vi "Begin.vi"(8 "error in":errorcluster) -> (0 "error out":errorcluster)   [LabVIEW 2019]
doc: "Called before other user functions, this VI is expected to open initial I/O refnums, load in file data, and do all program initialization. Notice that the <B>error out</B> terminal is simply used for data flow. Wiring it to other structures or subVIs ensures that this VI runs first."
uses:
  <vilib>/Rock Robotics/WPI/DriverStation/WPI_DriverStationRobotMode2.ctl
  <vilib>/Rock Robotics/WPI/Joystick/WPI_JoystickDeviceEnum.ctl
  <vilib>/Rock Robotics/WPI/Solenoid/WPI_SolenoidChannel.ctl
  <vilib>/Rock Robotics/SystemInterfaces/spilib/spi_bus.ctl
  <vilib>/Rock Robotics/WPI/ThirdParty/Phoenix-LabVIEW/Motor Controller/Controls/CTRE_Phoenix_MotorControl_NeutralMode.ctl
  <vilib>/Playing With Fusion Inc/Playing With Fusion Lib for FRC/PWF_ToF_LabVIEW/Public/TypeDefs/PwF_ToF_RangingMode.ctl
  <vilib>/Rock Robotics/WPI/ThirdParty/Phoenix-LabVIEW/Motor Controller/Controls/CTRE_Phoenix_MotorControl_ControlMode.ctl
  <vilib>/Rock Robotics/SystemInterfaces/i2clib/i2c_bus.ctl
  Robot Global Data.vi
  <vilib>/Rock Robotics/Network Tables/NT Write String Array.vi
  <vilib>/Rock Robotics/Network Tables/NT Read Number.vi
  <vilib>/Rock Robotics/WPI/Solenoid/WPI_SolenoidOpenSingle.vi
  <vilib>/Rock Robotics/WPI/Gyro/WPI_GyroXRS450_SPI_Open.vi
  GlobalRefnum.vi
  <vilib>/Rock Robotics/WPI/RobotDrive/WPI_RobotDriveOpen2MotorWithExistingMotors.vi
  <vilib>/Playing With Fusion Inc/Playing With Fusion Lib for FRC/PWF_ToF_LabVIEW/PwF_ToF.lvlib
panel:
  in  "F Shooter":dbl=0.049
  in  "D Shooter":dbl
  in  "I Shooter":dbl
  in  "P Shooter":dbl=0.1
  # "Shooter PID"
  # "10"
  # "1"
  # "3"
  # "5"
  # "6"
  # "7"
  # "8"
  # "9"
  # "2"
  # "4"
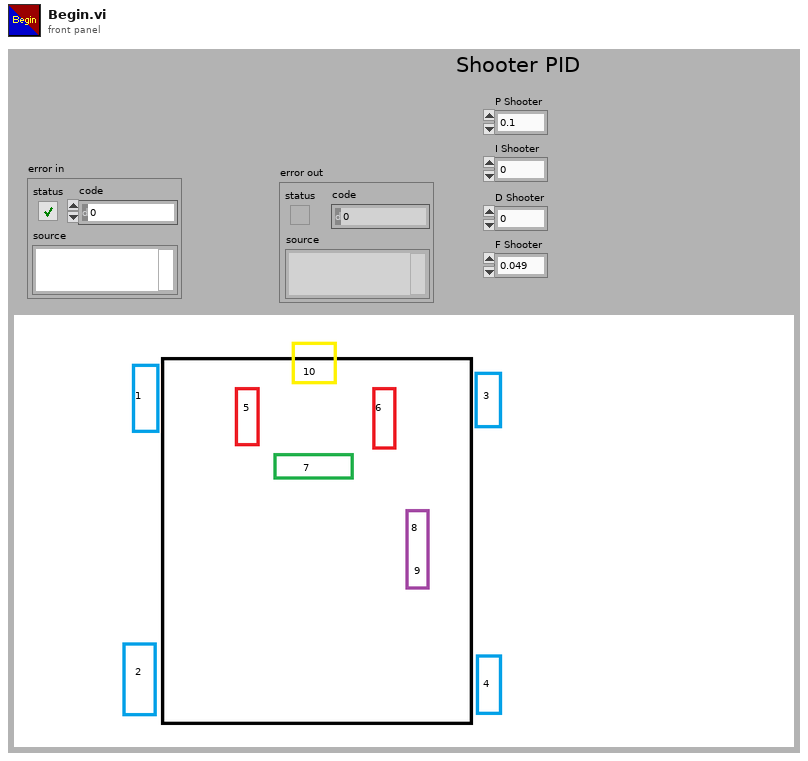
[diagram p1: front panel]
types:
  T1 = typedef "i2c_bus.ctl" = enum16{"I2C On-Board", "I2C MXP", "Invalid"}
  T2 = typedef "PlayingWithFusionLib.lvlib/PwF_ToF.lvlib/PwF_ToF_RangingMode.ctl" = enum16{"Short", "Medium", "Long"}
  T3 = typedef "CTRE_Phoenix_MotorControl_ControlMode.ctl" = u16
  T4 = typedef "WPI_SolenoidChannel.ctl" = enum8{"Solenoid 0", "Solenoid 1", "Solenoid 2", "Solenoid 3", "Solenoid 4", "Solenoid 5", "Solenoid 6", "Solenoid 7", "Invalid"}
  T5 = typedef "CTRE_Phoenix_MotorControl_NeutralMode.ctl" = enum8{"EEPROMSetting", "Override to Coast", "Override to Brake"}
  T6 = typedef "spi_bus.ctl" = enum16{"SPI On-Board, CS0", "SPI On-Board, CS1", "SPI On-Board, CS2", "SPI On-Board, CS3", "SPI MXP", "Invalid"}
  T7 = cluster{"2offsetAngle H":dbl, "2offsetAngle V":dbl, "2area":dbl, "2skew":dbl}
  T8 = cluster{"offsetAngle H":dbl, "offsetAngle V":dbl, "area":dbl, "skew":dbl}
  T9 = typedef "WPI_JoystickDeviceEnum.ctl" = enum16{"USB 0", "USB 1", "USB 2", "USB 3", "USB 4", "USB 5"}
  T10 = typedef "WPI_DriverStationRobotMode2.ctl" = enum16{"Autonomous Disabled", "Autonomous Enabled", "Teleop Disabled", "Teleop Enabled", "Disconnected", "Finish", "Test Disabled", "Test Enabled", "Emergency Stopped"}
  T11 = typedef "WPI_JoystickDevRef.ctl" = cluster{"Device":T9}
  T12 = typedef "WPI_MotorControlDeviceRef.ctl" = cluster{"DeviceStatus":errorcluster, "Type":T13, "PWM":cluster{"PWM Channel":T14, "DeadBand":T15}, "CAN":cluster{"Device Number":u8, "SetOutput VI Ref":variant, "GetOutput VI Ref":variant, "Enable VI Ref":variant, "Disable VI Ref":variant, "Data":variant}, "Invert":bool, "DIO PWM":cluster{"PWM \"Enable\" Channel":T14, "DIOChannel":T16, "PWM Rate":dbl}}
  T13 = typedef "WPI_MotorControlType.ctl" = enum16{"PWM", "CAN", "DIO PWM"}
  T14 = typedef "FPGA_DIOPWMChannel.ctl" = enum8{"PWM 0", "PWM 1", "PWM 2", "PWM 3", "PWM 4", "PWM 5", "PWM 6", "PWM 7", "PWM 8", "PWM 9", "PWM MXP 0", "PWM MXP 1", "PWM MXP 2", "PWM MXP 3", "PWM MXP 4", "PWM MXP 5", "PWM MXP 6", "PWM MXP 7", "PWM MXP 8", "PWM MXP 9", "Invalid"}
  T15 = typedef "WPI_PWMDeadband.ctl" = cluster{"Name":string, "maxPositivePwm":i32, "minPositivePwm":i32, "centerPwm":i32, "maxNegativePwm":i32, "minNegativePwm":i32, "angularRange":u16}
  T16 = typedef "FPGA_DIOChannel.ctl" = enum8{"DIO 0", "DIO 1", "DIO 2", "DIO 3", "DIO 4", "DIO 5", "DIO 6", "DIO 7", "DIO 8", "DIO 9", "DIO MXP 0", "DIO MXP 1", "DIO MXP 2", "DIO MXP 3", "DIO MXP 4", "DIO MXP 5", "DIO MXP 6", "DIO MXP 7", "DIO MXP 8", "DIO MXP 9", "DIO MXP 10", "DIO MXP 11", "DIO MXP 12", "DIO MXP 13", "DIO MXP 14", "DIO MXP 15", "SPI Port CS1", "SPI Port CS2", "SPI Port CS3", "SPI Port MISO", "SPI Port MOSI", "Invalid"}
  T17 = typedef "WPI_I2CDevRef.ctl" = cluster{"DevStatus":errorcluster, "Device Address":u8, "Handle":i32, "I2C Bus":T1}
  T18 = typedef "WPI_RobotDriveDevRef.ctl" = cluster{"DevStatus":errorcluster, "Motors[]":T12[], "Square Inputs":bool, "Max Output":dbl}
  T19 = typedef "WPI_CompressorDevRef.ctl" = cluster{"DevStatus":errorcluster, "Pneumatics Control Module":u8}
  T20 = typedef "WPI_SolenoidDevRef.ctl" = cluster{"DevStatus":errorcluster, "Pneumatics Control Module":u8, "Forward Solenoid Channel":T4, "Reverse Solenoid Channel":T4}
  T21 = typedef "WPI_GyroDevRef.ctl" = cluster{"DevStatus":errorcluster, "Analog Channel":T22, "Gain (VoltsPerDegree/Second)":dbl, "Gyro Type":enum16{"Analog", "XRS450"}, "Handle":i32, "SPI Bus":T6, "Device Found":bool, "Sample Rate":dbl, "Calibrate On Open":bool, "Offset":dbl}
  T22 = typedef "FPGA_AIChannel.ctl" = enum8{"AI 0", "AI 1", "AI 2", "AI 3", "AI MXP 0", "AI MXP 1", "AI MXP 2", "AI MXP 3", "Invalid"}
  T23 = typedef "PlayingWithFusionLib.lvlib/PwF_ToF.lvlib/PwF_ToF_DevRef.ctl" = cluster{"DeviceStatus":errorcluster, "Device Number":u8, "Handle":u64, "Library Path":path}
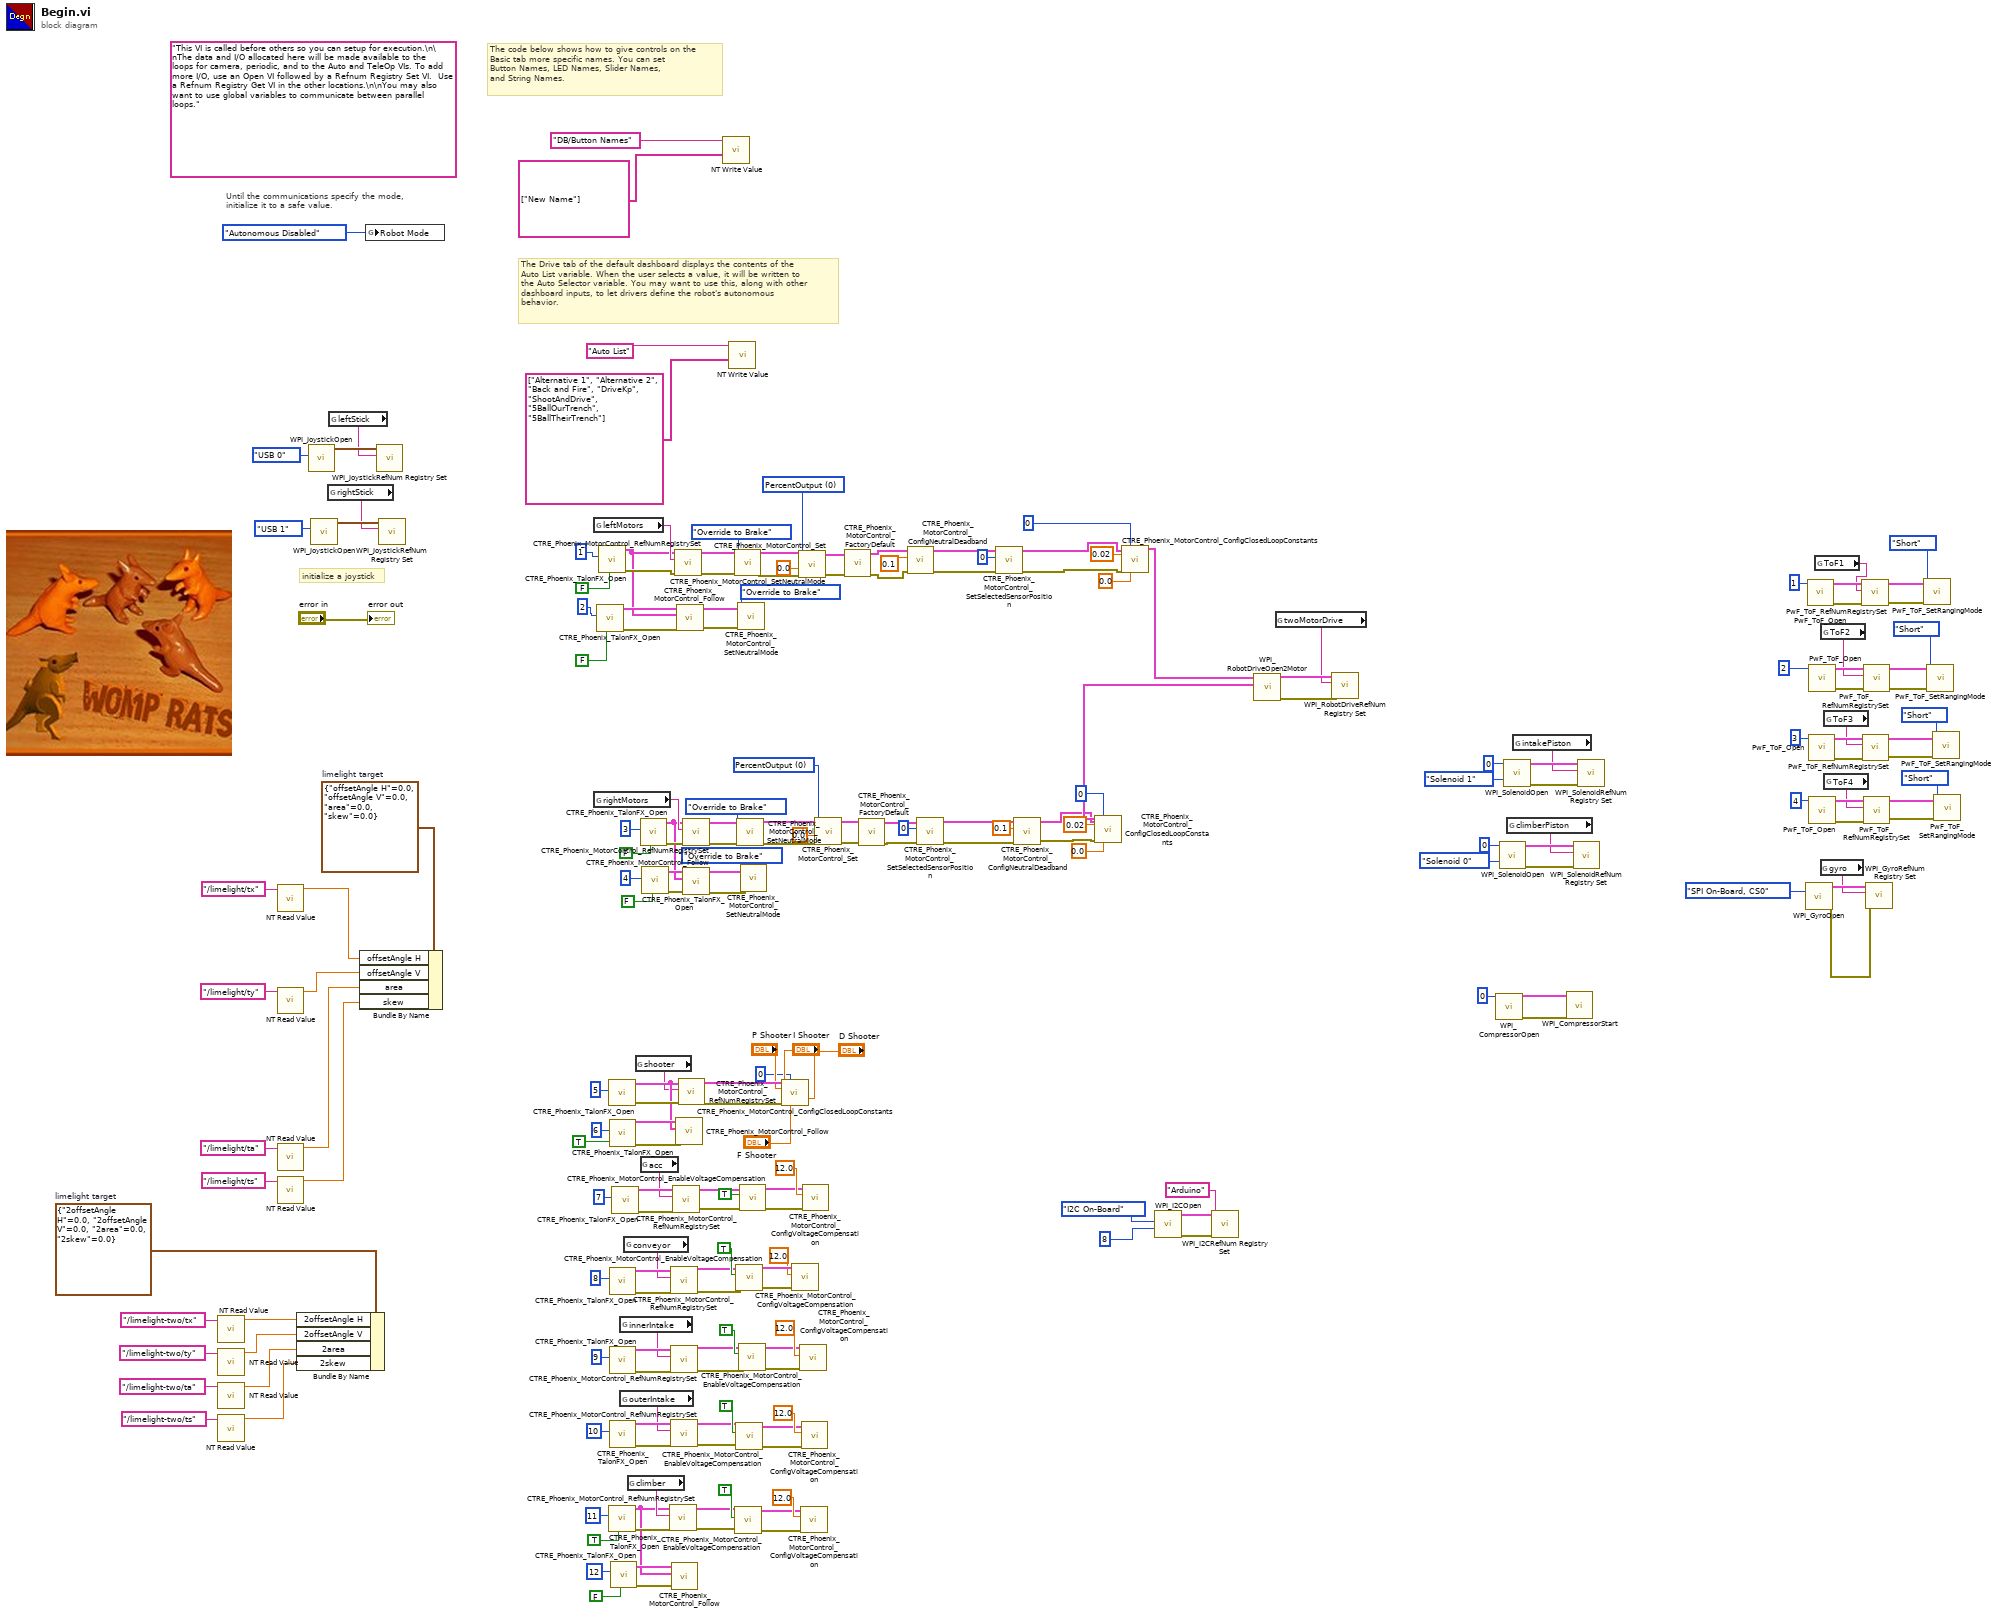
[diagram p0: block diagram]
diagram:
  w24 = T3 0 items=["PercentOutput"=0, "Position"=1, "Velocity"=2, "Current"=3, "Follower"=5, "MotionProfile"=6, "MotionMagic"=7, "MotionProfileArc"=10, "Disabled"=15] ("Control Mode")
  w34 = T3 0 items=["PercentOutput"=0, "Position"=1, "Velocity"=2, "Current"=3, "Follower"=5, "MotionProfile"=6, "MotionMagic"=7, "MotionProfileArc"=10, "Disabled"=15] ("Control Mode")
  w168 = T7 {"2offsetAngle H"=0.0, "2offsetAngle V"=0.0, "2area"=0.0, "2skew"=0.0}  # limelight target
  w203 = T8 {"offsetAngle H"=0.0, "offsetAngle V"=0.0, "area"=0.0, "skew"=0.0}  # limelight target
  (unwired) "This VI is called before others so you can setup for execution.\n\nThe data and I/O allocated here will be made available to the loops for camera, periodic, and to the Auto and TeleOp VIs. To add more I/O, use an Open VI followed by a Refnum Registry Set VI.  Use a Refnum Registry Get VI in the other locations.\n\nYou may also want to use global variables to communicate between parallel loops."
  # "The Drive tab of the default dashboard displays the contents of the\nAuto List variable. When the user selects a value, it will be written to\nthe Auto Selector variable. You may want to use this, along with other\ndashboard inputs, to let drivers define the robot's autonomous\nbehavior."
  # "The code below shows how to give controls on the\nBasic tab more specific names. You can set\nButton Names, LED Names, Slider Names,\nand String Names."
  # "initialize a joystick"
  # "Until the communications specify the mode,\ninitialize it to a safe value."
  n1 = call-poly <vilib>:"NT Read Value.vi"("Name"="/limelight-two/tx") -> ("Numeric"=w172:dbl)  [unwired: 9 in, 1 out]
  n2 = call-poly <vilib>:"NT Read Value.vi"("Name"="/limelight-two/ty") -> ("Numeric"=w171:dbl)  [unwired: 9 in, 1 out]
  n3 = call-poly <vilib>:"NT Read Value.vi"("Name"="/limelight-two/ta") -> ("Numeric"=w170:dbl)  [unwired: 9 in, 1 out]
  n4 = call-poly <vilib>:"NT Read Value.vi"("Name"="/limelight-two/ts") -> ("Numeric"=w169:dbl)  [unwired: 9 in, 1 out]
  n5 = call-poly <vilib>:"NT Read Value.vi"("Name"="/limelight/tx") -> ("Numeric"=w202:dbl)  [unwired: 9 in, 1 out]
  n6 = call-poly <vilib>:"NT Read Value.vi"("Name"="/limelight/ty") -> ("Numeric"=w201:dbl)  [unwired: 9 in, 1 out]
  n7 = call-poly <vilib>:"NT Read Value.vi"("Name"="/limelight/ta") -> ("Numeric"=w200:dbl)  [unwired: 9 in, 1 out]
  n8 = call-poly <vilib>:"NT Read Value.vi"("Name"="/limelight/ts") -> ("Numeric"=w199:dbl)  [unwired: 9 in, 1 out]
  n9 = Bundle By Name(cluster=w168, "2offsetAngle H"=w172, "2offsetAngle V"=w171, "2area"=w170, "2skew"=w169) -> ()  [unwired: 1 out]
  n10 = call <vilib>:"WPI_JoystickOpen.vi"("JoystickDevice"=WPI_JoystickDeviceEnum."USB 0") -> ("JoystickDevRef"=w218:T11)  [unwired: 10 in]
  n11 = call <vilib>:"WPI_JoystickOpen.vi"("JoystickDevice"=WPI_JoystickDeviceEnum."USB 1") -> ("JoystickDevRef"=w210:T11)  [unwired: 10 in]
  n12 = global read "GlobalRefnum.vi" "rightStick"() -> (w208:string)
  n13 = global read "GlobalRefnum.vi" "leftStick"() -> (w211:string)
  n14 = Bundle By Name(cluster=w203, "offsetAngle H"=w202, "offsetAngle V"=w201, "area"=w200, "skew"=w199) -> ()  [unwired: 1 out]
  n15 = global write "Robot Global Data.vi" "Robot Mode"(WPI_DriverStationRobotMode2."Autonomous Disabled" ("Robot Mode")) -> ()
  n16 = call <vilib>:"WPI_JoystickRefNum Registry Set.vi"("refnum name"=w211, "JoystickDevRef"=w218) -> ()  [unwired: 8 in, 2 out]
  n17 = call <vilib>:"WPI_JoystickRefNum Registry Set.vi"("refnum name"=w208, "JoystickDevRef"=w210) -> ()  [unwired: 8 in, 2 out]
  n18 = global read "GlobalRefnum.vi" "leftMotors"() -> (w189:string)
  n19 = global read "GlobalRefnum.vi" "rightMotors"() -> (w193:string)
  n20 = call <vilib>:"CTRE_Phoenix_TalonFX_Open.vi"("Invert"=FALSE, "Device Number"=u8 2) -> ("error out"=w182:errorcluster, "CAN Talon SRX Ref"=w181:T12)  [unwired: 8 in]
  n21 = call <vilib>:"CTRE_Phoenix_TalonFX_Open.vi"("Invert"=FALSE, "Device Number"=u8 1) -> ("error out"=w183:errorcluster, "CAN Talon SRX Ref"=w121:T12)  [unwired: 8 in]
  n22 = call <vilib>:"CTRE_Phoenix_TalonFX_Open.vi"("Device Number"=u8 5) -> ("error out"=w119:errorcluster, "CAN Talon SRX Ref"=w114:T12)  [unwired: 9 in]
  n23 = call <vilib>:"CTRE_Phoenix_TalonFX_Open.vi"("Invert"=TRUE, "Device Number"=u8 11) -> ("error out"=w63:errorcluster, "CAN Talon SRX Ref"=w52:T12)  [unwired: 8 in]
  n24 = call <vilib>:"CTRE_Phoenix_TalonFX_Open.vi"("Invert"=TRUE, "Device Number"=u8 6) -> ("error out"=w115:errorcluster, "CAN Talon SRX Ref"=w116:T12)  [unwired: 8 in]
  n25 = call <vilib>:"CTRE_Phoenix_TalonFX_Open.vi"("Device Number"=u8 8) -> ("error out"=w105:errorcluster, "CAN Talon SRX Ref"=w106:T12)  [unwired: 9 in]
  n26 = call <vilib>:"CTRE_Phoenix_TalonFX_Open.vi"("Device Number"=u8 9) -> ("error out"=w101:errorcluster, "CAN Talon SRX Ref"=w102:T12)  [unwired: 9 in]
  n27 = call <vilib>:"CTRE_Phoenix_TalonFX_Open.vi"("Device Number"=u8 10) -> ("error out"=w90:errorcluster, "CAN Talon SRX Ref"=w91:T12)  [unwired: 9 in]
  n28 = call <vilib>:"CTRE_Phoenix_TalonFX_Open.vi"("Invert"=FALSE, "Device Number"=u8 12) -> ("error out"=w54:errorcluster, "CAN Talon SRX Ref"=w55:T12)  [unwired: 8 in]
  n29 = call <vilib>:"CTRE_Phoenix_TalonFX_Open.vi"("Device Number"=u8 7) -> ("error out"=w109:errorcluster, "CAN Talon SRX Ref"=w110:T12)  [unwired: 9 in]
  n30 = global read "GlobalRefnum.vi" "innerIntake"() -> (w100:string)
  n31 = global read "GlobalRefnum.vi" "outerIntake"() -> (w89:string)
  n32 = global read "GlobalRefnum.vi" "conveyor"() -> (w104:string)
  n33 = global read "GlobalRefnum.vi" "climber"() -> (w62:string)
  n34 = global read "GlobalRefnum.vi" "shooter"() -> (w113:string)
  n35 = call <vilib>:"CTRE_Phoenix_TalonFX_Open.vi"("Invert"=FALSE, "Device Number"=u8 3) -> ("error out"=w188:errorcluster, "CAN Talon SRX Ref"=w120:T12)  [unwired: 8 in]
  n36 = global read "GlobalRefnum.vi" "acc"() -> (w108:string)
  n37 = call <vilib>:"CTRE_Phoenix_TalonFX_Open.vi"("Invert"=FALSE, "Device Number"=u8 4) -> ("error out"=w184:errorcluster, "CAN Talon SRX Ref"=w185:T12)  [unwired: 8 in]
  n38 = call <vilib>:"CTRE_Phoenix_MotorControl_RefNumRegistrySet.vi"("error in (no error)"=w63, "refnum name"=w62, "PhoenixMotorControlDevRef"=w52) -> ("error out"=w59:errorcluster, "PhoenixMotorControlDevRef"=w60:T12)  [unwired: 7 in]
  n39 = call <vilib>:"CTRE_Phoenix_MotorControl_RefNumRegistrySet.vi"("error in (no error)"=w105, "refnum name"=w104, "PhoenixMotorControlDevRef"=w106) -> ("error out"=w84:errorcluster, "PhoenixMotorControlDevRef"=w83:T12)  [unwired: 7 in]
  n40 = call <vilib>:"CTRE_Phoenix_MotorControl_RefNumRegistrySet.vi"("error in (no error)"=w101, "refnum name"=w100, "PhoenixMotorControlDevRef"=w102) -> ("error out"=w80:errorcluster, "PhoenixMotorControlDevRef"=w81:T12)  [unwired: 7 in]
  n41 = call <vilib>:"CTRE_Phoenix_MotorControl_RefNumRegistrySet.vi"("error in (no error)"=w90, "refnum name"=w89, "PhoenixMotorControlDevRef"=w91) -> ("error out"=w77:errorcluster, "PhoenixMotorControlDevRef"=w78:T12)  [unwired: 7 in]
  n42 = call <vilib>:"CTRE_Phoenix_MotorControl_Follow.vi"("error in (no error)"=w54, "Master Controller to Follow"=w52, "PhoenixMotorControlDevRef"=w55) -> ()  [unwired: 7 in, 2 out]
  n43 = call <vilib>:"CTRE_Phoenix_MotorControl_RefNumRegistrySet.vi"("error in (no error)"=w109, "refnum name"=w108, "PhoenixMotorControlDevRef"=w110) -> ("error out"=w87:errorcluster, "PhoenixMotorControlDevRef"=w88:T12)  [unwired: 7 in]
  n44 = call <vilib>:"CTRE_Phoenix_MotorControl_RefNumRegistrySet.vi"("error in (no error)"=w183, "refnum name"=w189, "PhoenixMotorControlDevRef"=w121) -> ("error out"=w151:errorcluster, "PhoenixMotorControlDevRef"=w150:T12)  [unwired: 7 in]
  n45 = call <vilib>:"CTRE_Phoenix_MotorControl_Follow.vi"("error in (no error)"=w115, "Master Controller to Follow"=w114, "PhoenixMotorControlDevRef"=w116) -> ()  [unwired: 7 in, 2 out]
  n46 = call <vilib>:"CTRE_Phoenix_MotorControl_Follow.vi"("error in (no error)"=w182, "Master Controller to Follow"=w121, "PhoenixMotorControlDevRef"=w181) -> ("error out"=w147:errorcluster, "PhoenixMotorControlDevRef"=w148:T12)  [unwired: 7 in]
  n47 = call <vilib>:"CTRE_Phoenix_MotorControl_RefNumRegistrySet.vi"("error in (no error)"=w119, "refnum name"=w113, "PhoenixMotorControlDevRef"=w114) -> ("error out"=w98:errorcluster, "PhoenixMotorControlDevRef"=w99:T12)  [unwired: 7 in]
  n48 = call <vilib>:"CTRE_Phoenix_MotorControl_RefNumRegistrySet.vi"("error in (no error)"=w188, "refnum name"=w193, "PhoenixMotorControlDevRef"=w120) -> ("error out"=w144:errorcluster, "PhoenixMotorControlDevRef"=w145:T12)  [unwired: 7 in]
  n49 = call <vilib>:"CTRE_Phoenix_MotorControl_Follow.vi"("error in (no error)"=w184, "Master Controller to Follow"=w120, "PhoenixMotorControlDevRef"=w185) -> ("error out"=w142:errorcluster, "PhoenixMotorControlDevRef"=w143:T12)  [unwired: 7 in]
  n50 = call-poly <vilib>:"NT Write Value.vi"("String Array"=string[] ["New Name"], "Name"="DB/Button Names") -> ()  [unwired: 9 in, 1 out]
  n51 = call-poly <vilib>:"NT Write Value.vi"("String Array"=string[] ["Alternative 1", "Alternative 2", "Back and Fire", "DriveKp", "ShootAndDrive", "5BallOurTrench", "5BallTheirTrench"], "Name"="Auto List") -> ()  [unwired: 9 in, 1 out]
  n52 = call <vilib>:"CTRE_Phoenix_MotorControl_SetNeutralMode.vi"("error in (no error)"=w151, "Motor Control Neutral Mode"=CTRE_Phoenix_MotorControl_NeutralMode."Override to Brake", "PhoenixMotorControlDevRef"=w150) -> ("error out"=w35:errorcluster, "PhoenixMotorControlDevRef"=w36:T12)  [unwired: 7 in]
  n53 = call <vilib>:"CTRE_Phoenix_MotorControl_EnableVoltageCompensation.vi"("error in (no error)"=w59, "Enable Voltage Compensation?"=TRUE, "PhoenixMotorControlDevRef"=w60) -> ("error out"=w56:errorcluster, "PhoenixMotorControlDevRef"=w57:T12)  [unwired: 7 in]
  n54 = call <vilib>:"CTRE_Phoenix_MotorControl_EnableVoltageCompensation.vi"("error in (no error)"=w84, "Enable Voltage Compensation?"=TRUE, "PhoenixMotorControlDevRef"=w83) -> ("error out"=w75:errorcluster, "PhoenixMotorControlDevRef"=w76:T12)  [unwired: 7 in]
  n55 = call <vilib>:"CTRE_Phoenix_MotorControl_EnableVoltageCompensation.vi"("error in (no error)"=w77, "Enable Voltage Compensation?"=TRUE, "PhoenixMotorControlDevRef"=w78) -> ("error out"=w68:errorcluster, "PhoenixMotorControlDevRef"=w69:T12)  [unwired: 7 in]
  n56 = call <vilib>:"CTRE_Phoenix_MotorControl_SetNeutralMode.vi"("error in (no error)"=w144, "Motor Control Neutral Mode"=CTRE_Phoenix_MotorControl_NeutralMode."Override to Brake", "PhoenixMotorControlDevRef"=w145) -> ("error out"=w30:errorcluster, "PhoenixMotorControlDevRef"=w31:T12)  [unwired: 7 in]
  n57 = call <vilib>:"CTRE_Phoenix_MotorControl_SetNeutralMode.vi"("error in (no error)"=w147, "Motor Control Neutral Mode"=CTRE_Phoenix_MotorControl_NeutralMode."Override to Brake", "PhoenixMotorControlDevRef"=w148) -> ()  [unwired: 7 in, 2 out]
  n58 = call <vilib>:"CTRE_Phoenix_MotorControl_EnableVoltageCompensation.vi"("error in (no error)"=w80, "Enable Voltage Compensation?"=TRUE, "PhoenixMotorControlDevRef"=w81) -> ("error out"=w71:errorcluster, "PhoenixMotorControlDevRef"=w72:T12)  [unwired: 7 in]
  n59 = call <vilib>:"CTRE_Phoenix_MotorControl_EnableVoltageCompensation.vi"("error in (no error)"=w87, "Enable Voltage Compensation?"=TRUE, "PhoenixMotorControlDevRef"=w88) -> ("error out"=w65:errorcluster, "PhoenixMotorControlDevRef"=w66:T12)  [unwired: 7 in]
  n60 = call <vilib>:"CTRE_Phoenix_MotorControl_SetNeutralMode.vi"("error in (no error)"=w142, "Motor Control Neutral Mode"=CTRE_Phoenix_MotorControl_NeutralMode."Override to Brake", "PhoenixMotorControlDevRef"=w143) -> ()  [unwired: 7 in, 2 out]
  n61 = call <vilib>:"CTRE_Phoenix_MotorControl_ConfigClosedLoopConstants.vi"("PhoenixMotorControlDevRef"=w99, "slotIdx"=0, "P"="P Shooter", "I"="I Shooter", "D"="D Shooter", "error in (no error)"=w98, "F"="F Shooter") -> ()  [unwired: 7 in, 2 out]
  n62 = call <vilib>:"CTRE_Phoenix_MotorControl_ConfigVoltageCompensation.vi"("error in (no error)"=w75, "Saturation Voltage"=12.0, "PhoenixMotorControlDevRef"=w76) -> ()  [unwired: 7 in, 2 out]
  n63 = call <vilib>:"CTRE_Phoenix_MotorControl_Set.vi"("error in (no error)"=w35, "Output"=0.0, "Control Mode"=w34, "PhoenixMotorControlDevRef"=w36) -> ("error out"=w27:errorcluster, "PhoenixMotorControlDevRef"=w28:T12)  [unwired: 6 in]
  n64 = call <vilib>:"CTRE_Phoenix_MotorControl_ConfigVoltageCompensation.vi"("error in (no error)"=w71, "Saturation Voltage"=12.0, "PhoenixMotorControlDevRef"=w72) -> ()  [unwired: 7 in, 2 out]
  n65 = call <vilib>:"CTRE_Phoenix_MotorControl_ConfigVoltageCompensation.vi"("error in (no error)"=w56, "Saturation Voltage"=12.0, "PhoenixMotorControlDevRef"=w57) -> ()  [unwired: 7 in, 2 out]
  n66 = call <vilib>:"CTRE_Phoenix_MotorControl_ConfigVoltageCompensation.vi"("error in (no error)"=w68, "Saturation Voltage"=12.0, "PhoenixMotorControlDevRef"=w69) -> ()  [unwired: 7 in, 2 out]
  n67 = call <vilib>:"CTRE_Phoenix_MotorControl_ConfigVoltageCompensation.vi"("error in (no error)"=w65, "Saturation Voltage"=12.0, "PhoenixMotorControlDevRef"=w66) -> ()  [unwired: 7 in, 2 out]
  n68 = call <vilib>:"CTRE_Phoenix_MotorControl_Set.vi"("error in (no error)"=w30, "Output"=0.0, "Control Mode"=w24, "PhoenixMotorControlDevRef"=w31) -> ("error out"=w29:errorcluster, "PhoenixMotorControlDevRef"=w32:T12)  [unwired: 6 in]
  n69 = call <vilib>:"CTRE_Phoenix_MotorControl_FactoryDefault.vi"("error in"=w27, "PhoenixMotorControlDevRef"=w28) -> ("error out"=w26:errorcluster, "PhoenixMotorControlDevRef"=w25:T12)  [unwired: 8 in]
  n70 = call <vilib>:"CTRE_Phoenix_MotorControl_FactoryDefault.vi"("error in"=w29, "PhoenixMotorControlDevRef"=w32) -> ("error out"=w16:errorcluster, "PhoenixMotorControlDevRef"=w15:T12)  [unwired: 8 in]
  n71 = call <vilib>:"CTRE_Phoenix_MotorControl_ConfigNeutralDeadband.vi"("error in (no error)"=w26, "Percent Deadband"=0.1, "PhoenixMotorControlDevRef"=w25) -> ("error out"=w21:errorcluster, "PhoenixMotorControlDevRef"=w22:T12)  [unwired: 7 in]
  n72 = call <vilib>:"CTRE_Phoenix_MotorControl_SetSelectedSensorPosition.vi"("error in (no error)"=w16, "New Sensor Position"=0, "PhoenixMotorControlDevRef"=w15) -> ("error out"=w17:errorcluster, "PhoenixMotorControlDevRef"=w18:T12)  [unwired: 7 in]
  n73 = call <vilib>:"CTRE_Phoenix_MotorControl_SetSelectedSensorPosition.vi"("error in (no error)"=w21, "New Sensor Position"=0, "PhoenixMotorControlDevRef"=w22) -> ("error out"=w19:errorcluster, "PhoenixMotorControlDevRef"=w20:T12)  [unwired: 7 in]
  n74 = call <vilib>:"CTRE_Phoenix_MotorControl_ConfigNeutralDeadband.vi"("error in (no error)"=w17, "Percent Deadband"=0.1, "PhoenixMotorControlDevRef"=w18) -> ("error out"=w39:errorcluster, "PhoenixMotorControlDevRef"=w40:T12)  [unwired: 7 in]
  n75 = call <vilib>:"CTRE_Phoenix_MotorControl_ConfigClosedLoopConstants.vi"("PhoenixMotorControlDevRef"=w40, "slotIdx"=0, "P"=0.02, "error in (no error)"=w39, "F"=0.0) -> ("PhoenixMotorControlDevRef"=w133:T12)  [unwired: 9 in, 1 out]
  n76 = call <vilib>:"CTRE_Phoenix_MotorControl_ConfigClosedLoopConstants.vi"("PhoenixMotorControlDevRef"=w20, "slotIdx"=0, "P"=0.02, "error in (no error)"=w19, "F"=0.0) -> ("PhoenixMotorControlDevRef"=w132:T12)  [unwired: 9 in, 1 out]
  n77 = call <vilib>:"WPI_I2COpen.vi"("Device Address"=u8 8, "I2C Bus"=i2c_bus."I2C On-Board") -> ("error out"=w5:errorcluster, "I2CDevRef"=w4:T17)  [unwired: 8 in]
  n78 = call <vilib>:"WPI_I2CRefNum Registry Set.vi"("error in (no error)"=w5, "refnum name"="Arduino", "I2CDevRef"=w4) -> ()  [unwired: 7 in, 2 out]
  n79 = call-poly <vilib>:"WPI_RobotDriveOpen2Motor.vi"("Right Motor Dev Ref"=w133, "Left Motor Dev Ref"=w132) -> ("error out"=w191:errorcluster, "RobotDriveDevRef"=w192:T18)  [unwired: 8 in]
  n80 = global read "GlobalRefnum.vi" "twoMotorDrive"() -> (w190:string)
  n81 = call <vilib>:"WPI_RobotDriveRefNum Registry Set.vi"("error in (no error)"=w191, "refnum name"=w190, "RobotDriveDevRef"=w192) -> ()  [unwired: 7 in, 2 out]
  n82 = call <vilib>:"WPI_CompressorOpen.vi"("Pneumatics Control Module (0)"=u8 0) -> ("CompressorDevRef"=w129:T19, "error out"=w128:errorcluster)  [unwired: 13 in]
  n83 = call-poly <vilib>:"WPI_SolenoidOpen.vi"("Solenoid Channel"=WPI_SolenoidChannel."Solenoid 0", "Pneumatics Control Module (0)"=u8 0) -> ("error out"=w123:errorcluster, "SolenoidDevRef"=w124:T20)  [unwired: 8 in]
  n84 = call-poly <vilib>:"WPI_SolenoidOpen.vi"("Solenoid Channel"=WPI_SolenoidChannel."Solenoid 1", "Pneumatics Control Module (0)"=u8 0) -> ("error out"=w195:errorcluster, "SolenoidDevRef"=w196:T20)  [unwired: 8 in]
  n85 = global read "GlobalRefnum.vi" "climberPiston"() -> (w122:string)
  n86 = global read "GlobalRefnum.vi" "intakePiston"() -> (w194:string)
  n87 = call <vilib>:"WPI_CompressorStart.vi"("error in (no error)"=w128, "CompressorDevRef"=w129) -> ()  [unwired: 8 in, 2 out]
  n88 = call <vilib>:"WPI_SolenoidRefNum Registry Set.vi"("error in (no error)"=w123, "refnum name"=w122, "SolenoidDevRef"=w124) -> ()  [unwired: 7 in, 2 out]
  n89 = call <vilib>:"WPI_SolenoidRefNum Registry Set.vi"("error in (no error)"=w195, "refnum name"=w194, "SolenoidDevRef"=w196) -> ()  [unwired: 7 in, 2 out]
  n90 = call-poly <vilib>:"WPI_GyroOpen.vi"("SPI Bus"=spi_bus."SPI On-Board, CS0") -> ("error out"=w154:errorcluster, "GyroDevRef"=w155:T21)  [unwired: 8 in, 1 out]
  n91 = call <vilib>:"PwF_ToF_Open.vi"("Device Number"=u8 1) -> ("error out"=w167:errorcluster, "PwFToFDevRef"=w166:T23)  [unwired: 9 in]
  n92 = call <vilib>:"PwF_ToF_Open.vi"("Device Number"=u8 3) -> ("error out"=w159:errorcluster, "PwFToFDevRef"=w158:T23)  [unwired: 9 in]
  n93 = call <vilib>:"PwF_ToF_Open.vi"("Device Number"=u8 2) -> ("error out"=w163:errorcluster, "PwFToFDevRef"=w162:T23)  [unwired: 9 in]
  n94 = call <vilib>:"PwF_ToF_Open.vi"("Device Number"=u8 4) -> ("error out"=w12:errorcluster, "PwFToFDevRef"=w11:T23)  [unwired: 9 in]
  n95 = global read "GlobalRefnum.vi" "ToF1"() -> (w165:string)
  n96 = global read "GlobalRefnum.vi" "gyro"() -> (w153:string)
  n97 = global read "GlobalRefnum.vi" "ToF2"() -> (w161:string)
  n98 = global read "GlobalRefnum.vi" "ToF3"() -> (w157:string)
  n99 = global read "GlobalRefnum.vi" "ToF4"() -> (w10:string)
  n100 = call <vilib>:"PwF_ToF_RefNumRegistrySet.vi"("error in (no error)"=w167, "refnum name"=w165, "PwFToFDevRefIn"=w166) -> ("error out"=w44:errorcluster, "PwFToFDevRefOut"=w45:T23)  [unwired: 7 in]
  n101 = call <vilib>:"PwF_ToF_RefNumRegistrySet.vi"("error in (no error)"=w159, "refnum name"=w157, "PwFToFDevRefIn"=w158) -> ("error out"=w41:errorcluster, "PwFToFDevRefOut"=w42:T23)  [unwired: 7 in]
  n102 = call <vilib>:"PwF_ToF_RefNumRegistrySet.vi"("error in (no error)"=w163, "refnum name"=w161, "PwFToFDevRefIn"=w162) -> ("error out"=w47:errorcluster, "PwFToFDevRefOut"=w49:T23)  [unwired: 7 in]
  n103 = call <vilib>:"PwF_ToF_RefNumRegistrySet.vi"("error in (no error)"=w12, "refnum name"=w10, "PwFToFDevRefIn"=w11) -> ("error out"=w6:errorcluster, "PwFToFDevRefOut"=w7:T23)  [unwired: 7 in]
  n104 = call <vilib>:"WPI_GyroRefNum Registry Set.vi"("error in (no error)"=w154, "refnum name"=w153, "GyroDevRef"=w155) -> ()  [unwired: 7 in, 2 out]
  n105 = call <vilib>:"PwF_ToF_SetRangingMode.vi"("error in"=w44, "RangingMode"=PwF_ToF_RangingMode."Short", "PwFToFDevRefIn"=w45) -> ()  [unwired: 7 in, 2 out]
  n106 = call <vilib>:"PwF_ToF_SetRangingMode.vi"("error in"=w47, "RangingMode"=PwF_ToF_RangingMode."Short", "PwFToFDevRefIn"=w49) -> ()  [unwired: 7 in, 2 out]
  n107 = call <vilib>:"PwF_ToF_SetRangingMode.vi"("error in"=w41, "RangingMode"=PwF_ToF_RangingMode."Short", "PwFToFDevRefIn"=w42) -> ()  [unwired: 7 in, 2 out]
  n108 = call <vilib>:"PwF_ToF_SetRangingMode.vi"("error in"=w6, "RangingMode"=PwF_ToF_RangingMode."Short", "PwFToFDevRefIn"=w7) -> ()  [unwired: 7 in, 2 out]
  "error out" <- "error in"
